vi "CVT2StaticReadTest.vi"() -> (3 "Unit Test Framework Results":T1)   [LabVIEW 2013, in "UnitTests.lvlib"]
uses:
  UnitTests.lvlib
  <vilib>/utf/common/utf_test_result_troll.ctl
  <vilib>/utf/common/utf_test_result.ctl
  <vilib>/utf/common/utf_test_result_failure.ctl
  <vilib>/utf/common/utf_test_comparison_operators.ctl
  <vilib>/utf/common/utf_vi_tag.ctl
  <vilib>/NI/Current Value Table/DataTypes/I32_Static Read.vi
  <vilib>/NI/Current Value Table/DataTypes/I32_Read.vi
  <vilib>/NI/Current Value Table/Type to Enum.vi
  <vilib>/NI/Current Value Table/DataTypes/I32_Type To Enum.vi
  <vilib>/NI/Current Value Table/FGVs/Tag Memory.vi
  <vilib>/NI/Current Value Table/Memory Block.vi
  <vilib>/NI/Current Value Table/DataTypes/I32_Memory Block.vi
  <vilib>/NI/Current Value Table/FGVs/CVT Globals.vi
  <vilib>/utf/NI_UnitTestFramework.lvlib
  <vilib>/NI/Current Value Table/Current Value Table.lvlib
panel:
  out "normal read":dbl
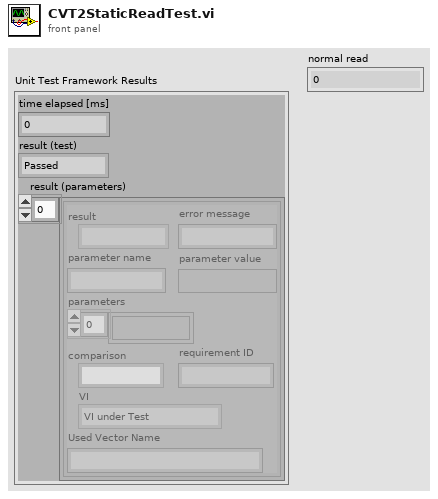
[diagram p1: front panel]
types:
  T1 = typedef "NI_UnitTestFramework.lvlib/utf_test_result_troll.ctl" = cluster{"time elapsed [ms]":u32, "result (test)":T2, "result (parameters)":T3[]}
  T2 = typedef "NI_UnitTestFramework.lvlib/utf_test_result.ctl" = enum16{"Passed", "Failed", "Error", "Skipped", "Not Processed"}
  T3 = typedef "NI_UnitTestFramework.lvlib/utf_test_result_failure.ctl" = cluster{"result":T2, "error message":string, "parameter name":string, "parameter value":variant, "parameters":variant[], "comparison":T4, "requirement ID":string, "VI":T5, "Used Vector Name":string}
  T4 = typedef "NI_UnitTestFramework.lvlib/utf_test_comparison_operators.ctl" = enum16{"=", "!=", ">", ">=", "<", "<=", "range", "symmetric tolerance", "asymmetric tolerance", "string contains", "string not contain", "array size", "string length", "array range", "by element", "array range (limit array)", "user-defined", "array contains", "array not contain", "vector length", "= (elm)", "!= (elm)", "= (case insensitive)", "!= (case insensitive)"}
  T5 = typedef "NI_UnitTestFramework.lvlib/utf_vi_tag.ctl" = enum16{"Setup VI", "VI under Test", "Teardown VI"}
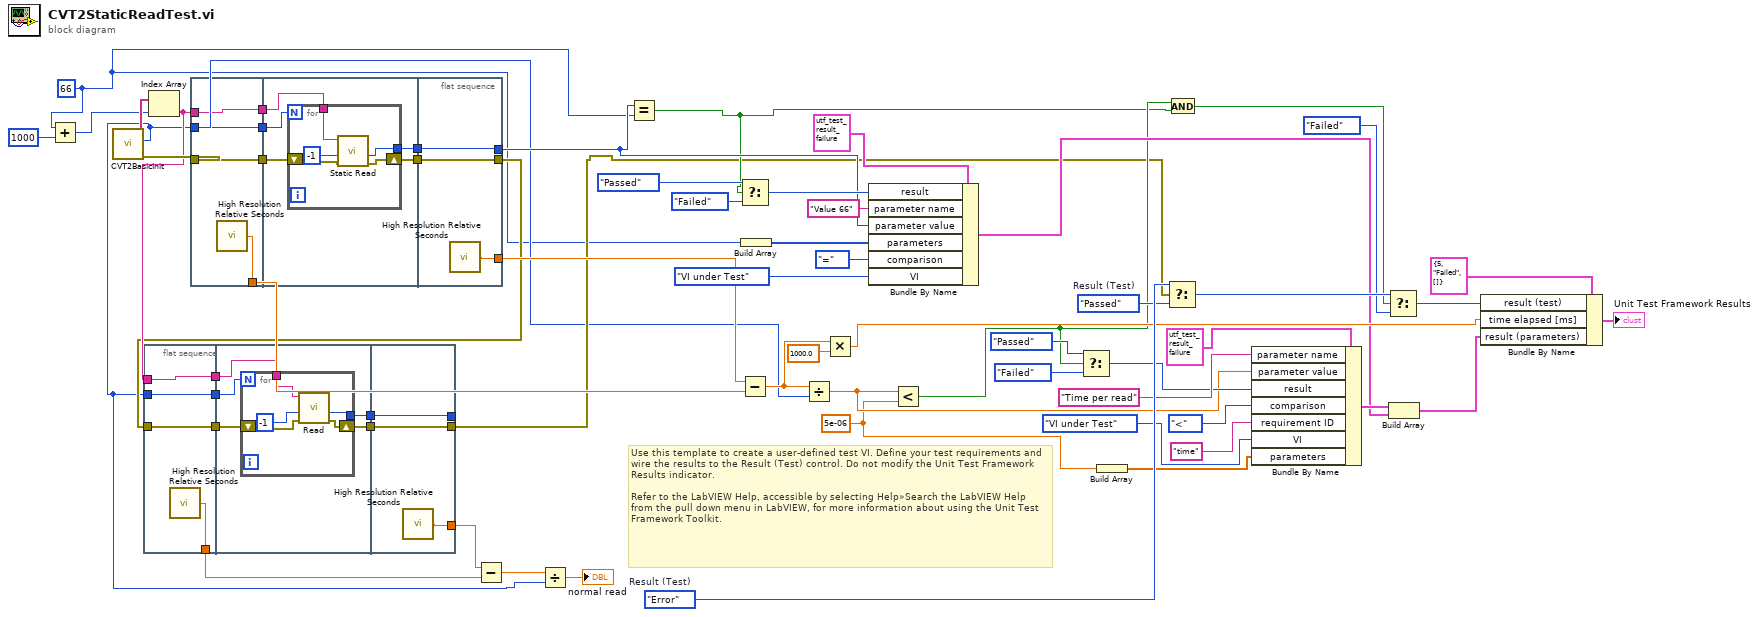
[diagram p0: block diagram]
diagram:
  w3 = 66 ("index")
  w36 = 5e-06 ("y")
  w56 = utf_test_result."Error"  # Result (Test)
  w55 = utf_test_result."Passed"  # Result (Test)
  # "Use this template to create a user-defined test VI. Define your test requirements and wire the results to the Result (Test) control. Do not modify the Unit Test Framework Results indicator. \n\nRefer to the LabVIEW Help, accessible by selecting Help»Search the LabVIEW Help from the pull down menu in LabVIEW, for more information about using the Unit Test Framework Toolkit."
  n1 = Add(x=w3, y=1000) -> (x+y=w2:i32)
  n2 = call "CVT2BasicInit.vi"() -> ("error out"=w20:errorcluster, "Tags per type out"=w5:i32, "names"=w19:string[])  [unwired: 9 in]
  n3 = flat-sequence {
    tunnel: [w65] -> w6
    tunnel: w10 -> [w64]
    tunnel: w5 -> [w63]
    tunnel: [w64] -> w16
    tunnel: [w63] -> w15
    tunnel: [w62] -> w14
    tunnel: w11 -> [w62]
    tunnel: w16 -> [w70]
    tunnel: [w69] -> w13
    tunnel: [w68] -> w12
    tunnel: w15 -> [w67]
    tunnel: w14 -> [w66]
    tunnel: [w78] -> w7
    tunnel: w13 -> [w77]
    tunnel: [w77] -> w9
    tunnel: [w76] -> _
    tunnel: w12 -> [w76]
    frame #0 {
      n4 = call <vilib>:"High Resolution Relative Seconds.vi"() -> ("relative seconds"=w65:dbl)
    }
    frame #1 {
      n5 = for {
        N: w67 -> [_]
        shift-right: [w71] -> w69
        shift-left: w70 -> [w75]
        tunnel: [w72] -> w68
        tunnel: w66 -> [w73]
        n6 = call-poly <vilib>:"Read.vi"("error in (no error)"=w75, "Default"=-1, "Tag Name"=w73) -> ("error out"=w71:errorcluster, "Value"=w72:i32)  [unwired: 7 in]
      }
    }
    frame #2 {
      n7 = call <vilib>:"High Resolution Relative Seconds.vi"() -> ("relative seconds"=w78:dbl)
    }
  }
  n8 = Index Array(array=w19, index=w2) -> (element=w11:string)
  n9 = flat-sequence {
    tunnel: [w82] -> w58
    tunnel: w20 -> [w81]
    tunnel: w5 -> [w80]
    tunnel: [w81] -> w50
    tunnel: [w80] -> w18
    tunnel: [w79] -> w17
    tunnel: w11 -> [w79]
    tunnel: w50 -> [w87]
    tunnel: [w86] -> w49
    tunnel: [w85] -> w31
    tunnel: w18 -> [w84]
    tunnel: w17 -> [w83]
    tunnel: [w95] -> w59
    tunnel: w49 -> [w94]
    tunnel: [w94] -> w10
    tunnel: [w93] -> w23
    tunnel: w31 -> [w93]
    frame #0 {
      n10 = call <vilib>:"High Resolution Relative Seconds.vi"() -> ("relative seconds"=w82:dbl)
    }
    frame #1 {
      n11 = for {
        N: w84 -> [_]
        shift-right: [w91] -> w86
        shift-left: w87 -> [w92]
        tunnel: [w90] -> w85
        tunnel: w83 -> [w89]
        n12 = call-poly <vilib>:"Static Read.vi"("error in (no error)"=w92, "Default"=-1, "Tag Name"=w89) -> ("error out"=w91:errorcluster, "Value"=w90:i32)  [unwired: 7 in]
      }
    }
    frame #2 {
      n13 = call <vilib>:"High Resolution Relative Seconds.vi"() -> ("relative seconds"=w95:dbl)
    }
  }
  n14 = Subtract(x=w7, y=w6) -> (x-y=w8:dbl)
  n15 = Divide(x=w8, y=w5) -> (x/y=→"normal read":dbl)
  n16 = Equal?(x=w23, y=w3) -> (x = y?=w22:bool)
  n17 = Select(t=utf_test_result."Passed" ("result"), s=w22, f=utf_test_result."Failed" ("result")) -> (s? t:f=w26:T2)
  n18 = Subtract(x=w59, y=w58) -> (x-y=w48:dbl)
  n19 = Build Array(w3) -> (w24:i32[])
  n20 = Divide(x=w48, y=w5) -> (x/y=w39:dbl)
  n21 = Multiply(x=w48, y=1000.0) -> (x*y=w51:dbl)
  n22 = Bundle By Name(cluster=T3 {"result"=enum."Passed", "error message"="", "parameter name"="", "parameter value"=variant, "parameters"=[], "comparison"=enum."=", "requirement ID"="", "VI"=enum."Setup VI", "Used Vector Name"=""} ("Unit Test Framework - result (parameters)"), "result"=w26, "parameter name"="Value 66", "parameter value"=w23, "parameters"=w24, "comparison"=utf_test_comparison_operators."=", "VI"=utf_vi_tag."VI under Test") -> (w34:T3)
  n23 = Less?(x=w39, y=w36) -> (x < y?=w32:bool)
  n24 = Select(t=utf_test_result."Passed" ("result"), s=w32, f=utf_test_result."Failed" ("result")) -> (s? t:f=w40:T2)
  n25 = Build Array(w36) -> (w35:dbl[])
  n26 = Select(t=w56, s=w9, f=w55) -> (s? t:f=w46:T2)
  n27 = And(x=w32, y=w22) -> (x .and. y?=w33:bool)
  n28 = Bundle By Name(cluster=T3 {"result"=enum."Passed", "error message"="", "parameter name"="", "parameter value"=variant, "parameters"=[], "comparison"=enum."=", "requirement ID"="", "VI"=enum."Setup VI", "Used Vector Name"=""} ("Unit Test Framework - result (parameters)"), "parameter name"="Time per read", "parameter value"=w39, "result"=w40, "comparison"=utf_test_comparison_operators."<", "requirement ID"="time", "VI"=utf_vi_tag."VI under Test", "parameters"=w35) -> (w54:T3)
  n29 = Select(t=w46, s=w33, f=utf_test_result."Failed") -> (s? t:f=w44:T2)
  n30 = Build Array(w54, w34) -> (w53:T3[])
  n31 = Bundle By Name(cluster=T1 {"time elapsed [ms]"=5, "result (test)"=enum."Failed", "result (parameters)"=[]} ("Unit Test Framework - Result"), "result (test)"=w44, "time elapsed [ms]"=w51, "result (parameters)"=w53) -> (→"Unit Test Framework Results":T1)
